vi "setView.vi"(10 "View.lvclass":refnum<class "View.lvclass">, 11 "Controller in":refnum<class "Controller.lvclass">) -> (3 "Controller out":refnum<class "Controller.lvclass">)   [LabVIEW 2016, in "Controller.lvclass"]
uses:
  Controller.lvclass
  View/View.lvclass
  Controller.lvclass/Controller.ctl
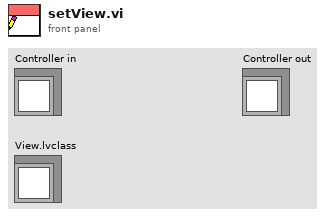
[diagram p1: front panel]
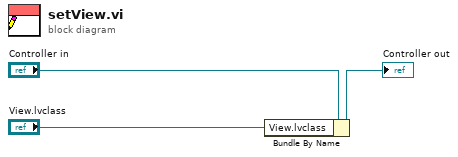
[diagram p0: block diagram]
diagram:
  n1 = Bundle By Name(cluster="Controller in", "View.lvclass"="View.lvclass") -> (→"Controller out":refnum<class "Controller.lvclass">)
